vi "load xml for traverse.vi"(8 "error in":errorcluster caption="错误输入（无错误）", 10 "Data in":T1, 11 "PanelRootNode 输入":refnum<class "PanelRootNode.lvclass"> caption="DNL_LabVIEW Object in") -> (0 "error out":errorcluster caption="错误输出", 1 "SubNodes":refnum<k20>[](array[refnum]), 2 "Data out":T1, 3 "PanelRootNode 输出":refnum<class "PanelRootNode.lvclass"> caption="DNL_LabVIEW Object out")   [LabVIEW 2016, in "PanelRootNode.lvclass"]
uses:
  PanelRootNode.lvclass
  C:/Users/CL/Desktop/ZcDAQprj0811/ZcDAQprj/Modules/DAQ-Display/PanelSplitToolkit/PanelLinkNode/PanelLinkNode.lvclass
  PanelLinkNode/PanelLinkNode.lvclass/PanelLinkNode.ctl
  <vilib>/xml/Close Reference(Node).vi
  PanelLinkNode/PanelLinkNode.lvclass
  <resource>/objmgr/DOMUserDefRef.rc
  <vilib>/xml/NI_XML.lvlib
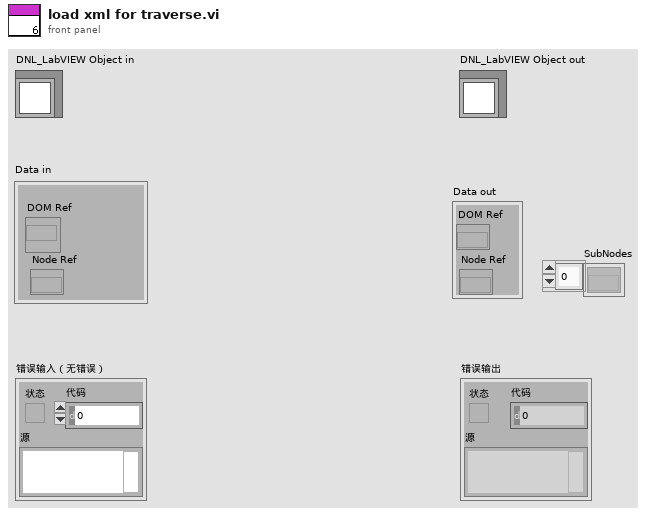
[diagram p1: front panel]
types:
  T1 = cluster{"DOM Ref":refnum<k20>, "Node Ref":refnum<k20>}
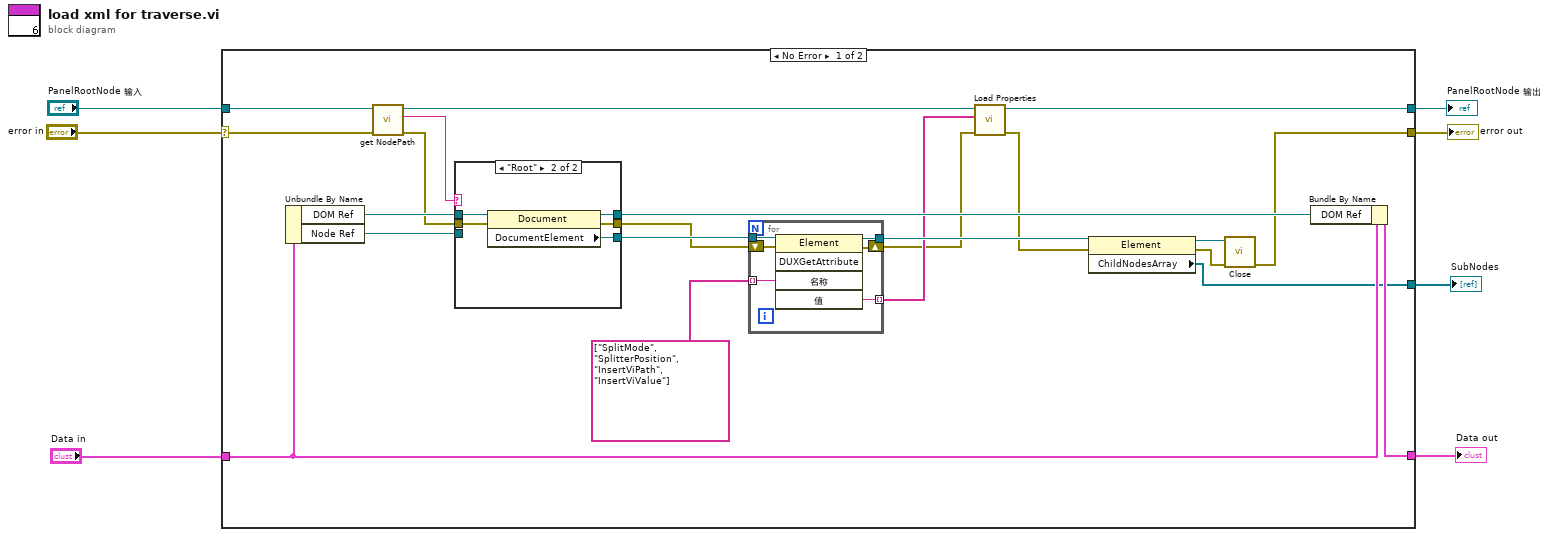
[diagram p0: block diagram]
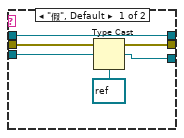
[diagram p2: hidden frame]
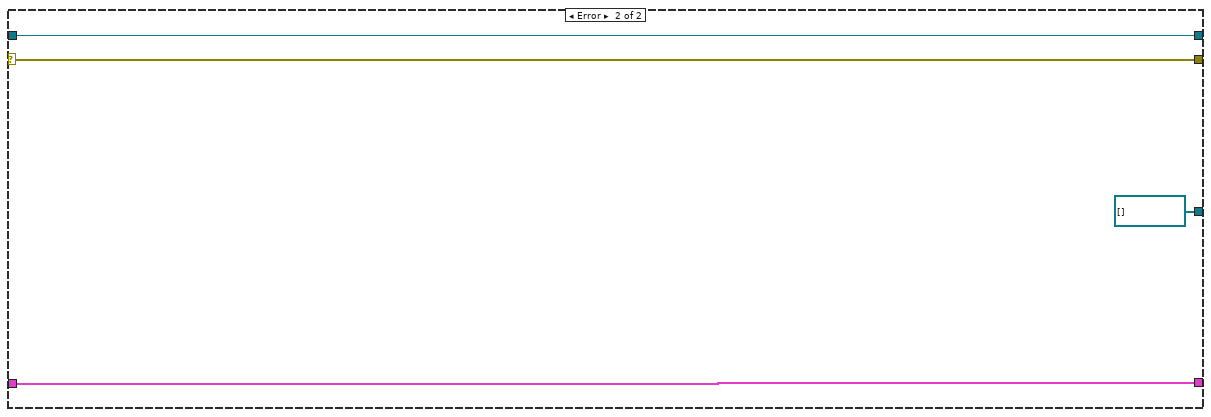
[diagram p3: hidden frame]
diagram:
  n1 = case shown="No Error" "error in" {
    selector: "error in" -> [w26 w49]
    tunnel: [w8 w49] -> w6
    tunnel: [w12 w48] -> w4
    tunnel: "PanelRootNode 输入" -> [w29 w48]
    tunnel: "Data in" -> [w28 w47]
    tunnel: [w27 w47] -> w2
    tunnel: [w16 refnum<k20>[] [] ("ChildNodesArray")] -> w1
    frame No Error {
      n2 = Unbundle By Name(w28) -> ("DOM Ref"=w25:refnum<k20>, "Node Ref"=w24:refnum<k20>)
      n3 = call "get NodePath.vi"("error in (no error)"=w26, "PanelLinkNode输入"=w29) -> ("error out"=w23:errorcluster, "NodePath"=w22:string, "PanelLinkNode输出"=w13:refnum<class "PanelRootNode.lvclass">)  [unwired: 7 in]
      n4 = case shown="\"Root\"" w22 {
        tunnel: [w40 w43] -> w18
        tunnel: w25 -> [w40 w45]
        tunnel: w24 -> [w38 _]
        tunnel: w23 -> [w36 w44]
        tunnel: [w37 w42] -> w20
        tunnel: [w36 w41] -> w14
        frame "假", Default {
          n5 = Type Cast(type=refnum<k20> refnum ("DocumentElement"), x=w38) -> (*(type *) &x=w37:refnum<k20>)
        }
        frame "Root" {
          n6 = property on="属性节点" class="Document"(reference=w45, error in=w44) -> (reference out=w43:refnum<k20>, error out=w41:errorcluster, "DocumentElement"=w42:refnum<k20>)
        }
      }
      n7 = for {
        tunnel: string[] ["SplitMode", "SplitterPosition", "InsertViPath", "InsertViValue"] -> [w35] mode=indexing
        tunnel: [w34] -> w11 mode=indexing
        tunnel: [w33] -> w21
        tunnel: w20 -> [w31]
        shift-right: [w32] -> w10
        shift-left: w14 -> [w30]
        n8 = invoke on="调用节点" class="Element" method="DUXGetAttribute"(reference=w31, error in=w30, "名称"=w35) -> (reference out=w33:refnum<k20>, error out=w32:errorcluster, "值"=w34:string)  [unwired: 2 in, 2 out]
      }
      n9 = call "Load Properties.vi"("error in"=w10, "Properties"=w11, "PanelRootNode 输入"=w13) -> ("error out"=w9:errorcluster, "PanelRootNode 输出"=w12:refnum<class "PanelRootNode.lvclass">)  [unwired: 7 in]
      n10 = property on="属性节点" class="Element"(reference=w21, error in=w9) -> (reference out=w19:refnum<k20>, error out=w17:errorcluster, "ChildNodesArray"=w16:refnum<k20>[])
      n11 = call-poly <vilib>:"Close.vi"("error in (no error)"=w17, "node"=w19) -> ("error out"=w8:errorcluster)  [unwired: 7 in]
      n12 = Bundle By Name(cluster=w28, "DOM Ref"=w18) -> (w27:T1)
    }
    frame Error {
    }
  }
  "error out" <- w6
  "PanelRootNode 输出" <- w4
  "Data out" <- w2
  "SubNodes" <- w1
